vi "SR SIM921 Set Curve Header.vi"(5 "Curve Data Format":T1(ring)=enum."LogLog", 7 "Curve ID String":string, 8 "Error In":errorcluster, 9 "Curve #":u32=1, 10 "Slot":T2(ring), 11 "VISA resource name":refnum<visa-resource-name>) -> (0 "Error Out":errorcluster, 3 "VISA resource name":refnum<visa-resource-name>)   [LabVIEW 2019]
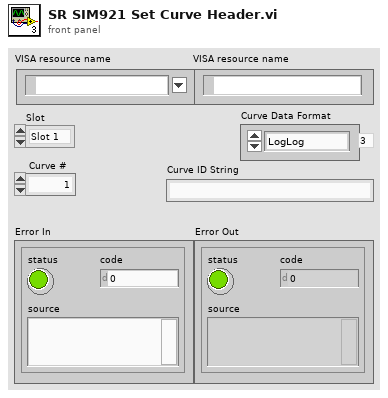
[diagram p1: front panel]
types:
  T1 = enum16{"Linear", "SemiLogT", "SemiLogR", "LogLog"}
  T2 = enum32{"Slot 1", "Slot 2", "Slot 3", "Slot 4", "Slot 5", "Slot 6", "Slot 7", "Slot 8"}
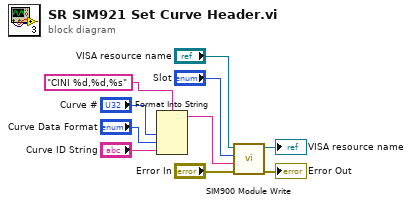
[diagram p0: block diagram]
diagram:
  n1 = Format Into String(format string="CINI %d,%d,%s", "Curve #", "Curve Data Format", "Curve ID String") -> (resulting string=w5:string)  [unwired: 2 in, 1 out]
  n2 = call "SIM900 Module Write.vi"("Error In"="Error In", "Query"=w5, "Slot"="Slot", "VISA Resource Name"="VISA resource name") -> ("Error Out"=→"Error Out":errorcluster, "dup VISA Session"=→"VISA resource name":refnum<visa-resource-name>)  [unwired: 6 in]
